vi "Read Header.vi"(7 "Linked List ID":string, 8 "error in (no error)":errorcluster, 10 "Header Name":string, 11 "Linked List in":refnum<class "Linked List.lvclass">) -> (0 "error out":errorcluster, 1 "found":bool, 2 "Header Value":string, 3 "Linked List out":refnum<class "Linked List.lvclass">)   [LabVIEW 2019, in "Linked Lists.lvlib" / "Linked List.lvclass"]
uses:
  <vilib>/gpm_packages/@cs/linked-list/Source/Linked List/Linked List/Linked List.lvclass
  <vilib>/gpm_packages/@cs/linked-list/Source/Linked List/Linked List Definition/Linked List Definition.lvclass
  <vilib>/gpm_packages/@cs/linked-list/Source/Linked List/Linked List/Linked List.lvclass/Linked List.ctl
  <vilib>/gpm_packages/@cs/lookup-table/Source/LookupTable/LookupTable.lvclass/LookupTable.ctl
  398019e9-15b1-4b22-94d3-e3336d36afb3.vi
  <vilib>/gpm_packages/@cs/lookup-table/Source/LookupTable/Read Table Reference.vi
  398019e9-15b1-4b22-94d3-e3336d36afb3.vi/1ffdd7f1-42f8-44d1-8aea-0d4919931cc6.vi
  <vilib>/gpm_packages/@cs/lookup-table/Source/LookupTable/LookupTable.lvclass
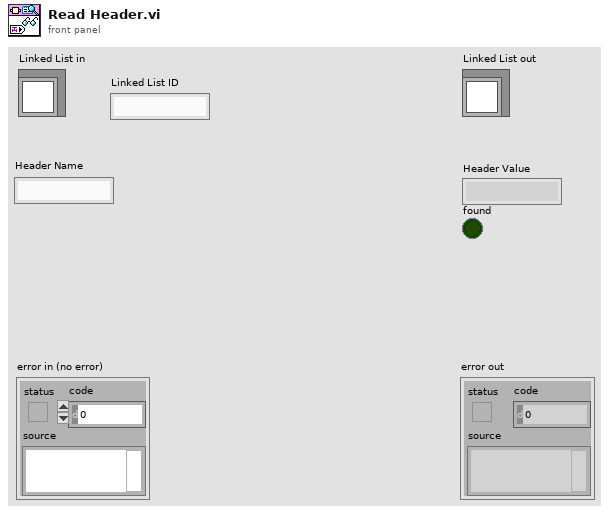
[diagram p1: front panel]
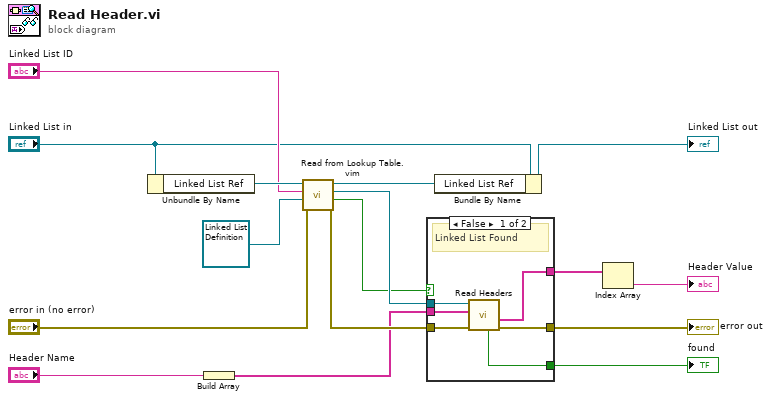
[diagram p0: block diagram]
diagram:
  n1 = Unbundle By Name("Linked List in") -> ("Linked List Ref"=w16:refnum<data-value>)
  n2 = Build Array("Header Name") -> (w5:string[])
  n3 = call "Read from Lookup Table.vim"("error in (no error)"="error in (no error)", "Type"=refnum<class "Linked List Definition.lvclass"> refnum ("Linked List.lvlib:Linked List Definition.lvclass"), "Item Name"="Linked List ID", "LookupTable Reference"=w16) -> ("error out"=w9:errorcluster, "Not Found?"=w4:bool, "Value"=w7:refnum<class "Linked List Definition.lvclass">, "LookupTable Reference Out"=w11:refnum<data-value>)  [unwired: 4 in]
  n4 = case shown="False" w4 {
    tunnel: w9 -> [w22 w23]
    tunnel: [w21 w23] -> w8
    tunnel: w7 -> [w20 _]
    tunnel: w5 -> [w19 _]
    tunnel: [w18 _] -> w3
    tunnel: [w17 _] -> w2
    frame False {
      # "Linked List Found"
      n5 = call <vilib>:"Read Headers.vi"("error in (no error)"=w22, "Header Names"=w19, "Linked List Definition in"=w20) -> ("error out"=w21:errorcluster, "Header Values"=w17:string[], "Found?"=w18:bool)  [unwired: 4 in, 2 out]
    }
    frame True {
      # "Linked List not found"
    }
  }
  "error out" <- w8
  "found" <- w3
  n6 = Bundle By Name(cluster="Linked List in", "Linked List Ref"=w11) -> (→"Linked List out":refnum<class "Linked List.lvclass">)
  n7 = Index Array(array=w2) -> (element=→"Header Value":string)  [unwired: 1 in]
